vi "Adj Controls Pos.vi"(0 "Decoration Ref Array":refnum<vi>[](array[refnum]), 2 "Panel Bounds":T1, 5 "Add Display Ref (Bool)":refnum<vi>, 7 "Remove Display Ref (Bool)":refnum<vi>, 9 "Exit (Bool)":refnum<vi>, 11 "Message (String)":refnum<vi>, 12 "Max Left (Bool)":refnum<vi>, 13 "Max Right (Bool)":refnum<vi>) -> ()   [LabVIEW 2016]
uses:
  <vilib>/Utility/miscctls.llb/LVRectTypeDef.ctl
panel:
  in  "Add Display":bool
  in  "Remove Display":bool
  # "Copyright (C) 2020 Edward S Allgeyer\n\nRedistribution and use in source and binary forms, with or without\nmodification, are permitted provided that the following conditions\nare met:\n\n1. Redistributions of source code must retain the above copyright\n   notice, this list of conditions and the following disclaimer.\n\n2. Redistributions in binary form must reproduce the above copyright\n   notice, this list of conditions and the following disclaimer in\n   the documentation and/or other materials provided with the\n   distribution.\n\n3. Neither the name of the copyright holder nor the names of its\n   contributors may be used to endorse or promote products derived\n   from this software without specific prior written permission.\n\nTHIS SOFTWARE IS PROVIDED BY THE COPYRIGHT HOLDERS AND CONTRIBUTORS\n\"AS IS\" AND ANY EXPRESS OR IMPLIED WARRANTIES, INCLUDING, BUT NOT\nLIMITED TO, THE IMPLIED WARRANTIES OF MERCHANTABILITY AND FITNESS\nFOR A PARTICULAR PURPOSE ARE DISCLAIMED. IN NO EVENT SHALL THE\nCOPYRIGHT HOLDER OR CONTRIBUTORS BE LIABLE FOR ANY DIRECT, INDIRECT,\nINCIDENTAL, SPECIAL, EXEMPLARY, OR CONSEQUENTIAL DAMAGES (INCLUDING,\nBUT NOT LIMITED TO, PROCUREMENT OF SUBSTITUTE GOODS OR SERVICES;\nLOSS OF USE, DATA, OR PROFITS; OR BUSINESS INTERRUPTION) HOWEVER\nCAUSED AND ON ANY THEORY OF LIABILITY, WHETHER IN CONTRACT, STRICT\nLIABILITY, OR TORT (INCLUDING NEGLIGENCE OR OTHERWISE) ARISING IN\nANY WAY OUT OF THE USE OF THIS SOFTWARE, EVEN IF ADVISED OF THE\nPOSSIBILITY OF SUCH DAMAGE."
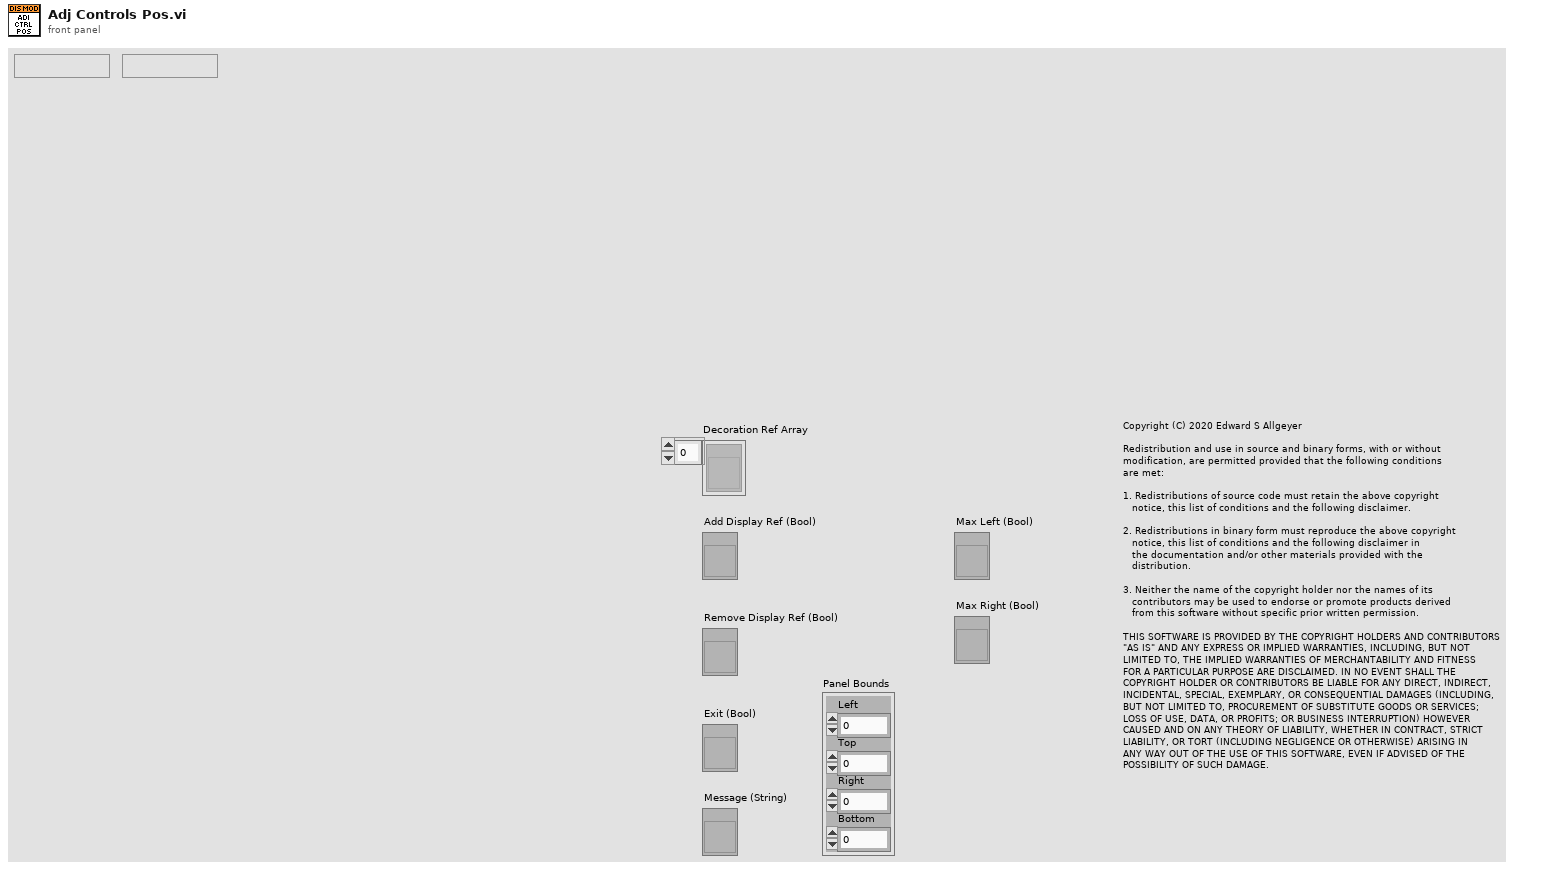
[diagram p1: front panel]
types:
  T1 = typedef "LVRectTypeDef.ctl" = cluster{"Left":i16, "Top":i16, "Right":i16, "Bottom":i16}
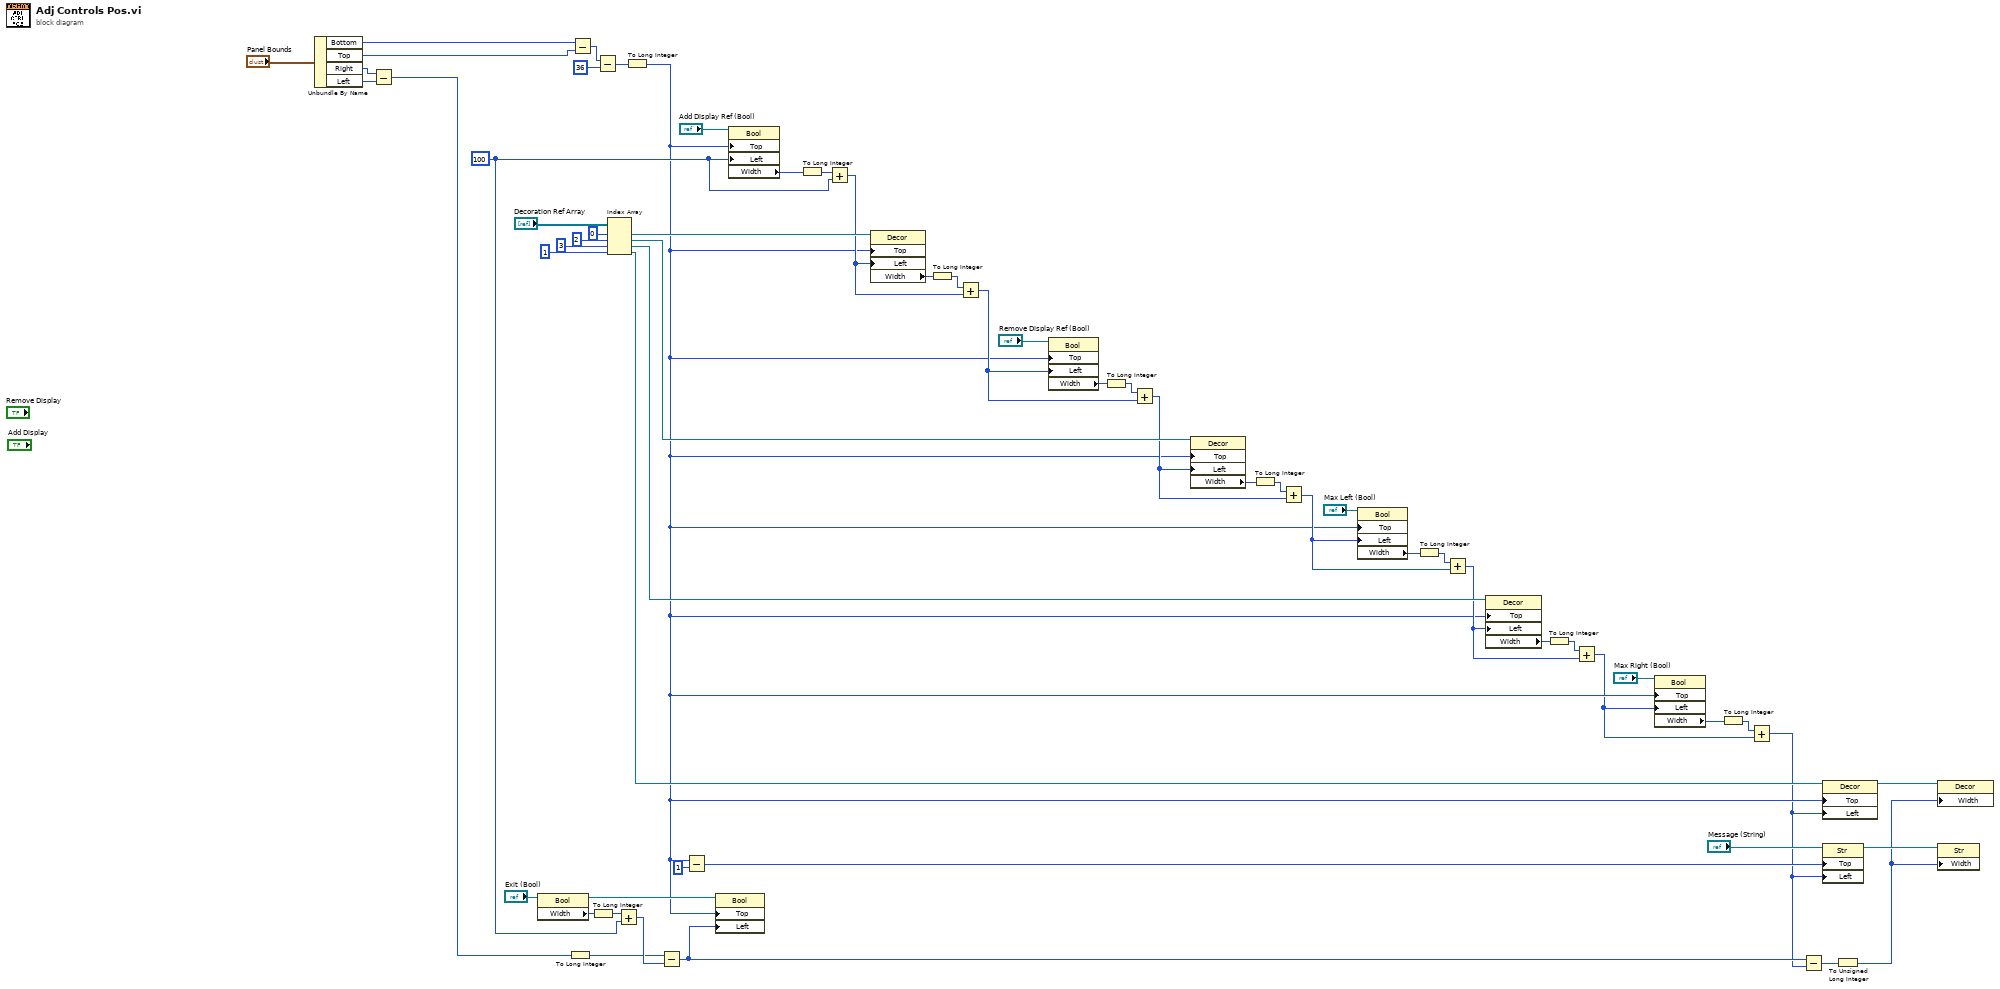
[diagram p0: block diagram]
diagram:
  w31 = 100 ("Position:Left")
  n1 = Unbundle By Name("Panel Bounds") -> ("Bottom"=w56:i16, "Top"=w55:i16, "Right"=w54:i16, "Left"=w53:i16)
  n2 = Subtract(x=w54, y=w53) -> (x-y=w29:i16)
  n3 = property class="Bool"(reference="Exit (Bool)") -> (reference out=w33:refnum<vi>, "Width"=w32:u32)  [unwired: 1 in, 1 out]
  n4 = To Long Integer(number=w29) -> (32bit integer=w27:i32)
  n5 = Subtract(x=w56, y=w55) -> (x-y=w59:i16)
  n6 = To Long Integer(number=w32) -> (32bit integer=w30:i32)
  n7 = Subtract(x=w59, y=i16 36) -> (x-y=w47:i16)
  n8 = Index Array(array="Decoration Ref Array", index #1=0 ("index"), index #2=2 ("index"), index #3=3 ("index"), index #4=1 ("index")) -> (element #1=w50:refnum<vi>, element #2=w17:refnum<vi>, element #3=w11:refnum<vi>, element #4=w19:refnum<vi>)
  n9 = Add(x=w30, y=w31) -> (x+y=w28:i32)
  n10 = To Long Integer(number=w47) -> (32bit integer=w5:i32)
  n11 = Subtract(x=w27, y=w28) -> (x-y=w24:i32)
  n12 = Subtract(x=w5, y=1) -> (x-y=w44:i32)
  n13 = property class="Bool"(reference=w33, "Top"=w5, "Left"=w24) -> ()  [unwired: 1 in, 2 out]
  n14 = property class="Bool"(reference="Add Display Ref (Bool)", "Top"=w5, "Left"=w31) -> ("Width"=w42:u32)  [unwired: 1 in, 2 out]
  n15 = To Long Integer(number=w42) -> (32bit integer=w41:i32)
  n16 = Add(x=w41, y=w31) -> (x+y=w36:i32)
  n17 = property class="Decor"(reference=w50, "Top"=w5, "Left"=w36) -> ("Width"=w40:u32)  [unwired: 1 in, 2 out]
  n18 = To Long Integer(number=w40) -> (32bit integer=w39:i32)
  n19 = Add(x=w39, y=w36) -> (x+y=w35:i32)
  n20 = property class="Bool"(reference="Remove Display Ref (Bool)", "Top"=w5, "Left"=w35) -> ("Width"=w37:u32)  [unwired: 1 in, 2 out]
  n21 = To Long Integer(number=w37) -> (32bit integer=w38:i32)
  n22 = Add(x=w38, y=w35) -> (x+y=w14:i32)
  n23 = property class="Decor"(reference=w17, "Top"=w5, "Left"=w14) -> ("Width"=w15:u32)  [unwired: 1 in, 2 out]
  n24 = To Long Integer(number=w15) -> (32bit integer=w16:i32)
  n25 = Add(x=w16, y=w14) -> (x+y=w10:i32)
  n26 = property class="Bool"(reference="Max Left (Bool)", "Top"=w5, "Left"=w10) -> ("Width"=w12:u32)  [unwired: 1 in, 2 out]
  n27 = To Long Integer(number=w12) -> (32bit integer=w13:i32)
  n28 = Add(x=w13, y=w10) -> (x+y=w7:i32)
  n29 = property class="Decor"(reference=w11, "Top"=w5, "Left"=w7) -> ("Width"=w8:u32)  [unwired: 1 in, 2 out]
  n30 = To Long Integer(number=w8) -> (32bit integer=w9:i32)
  n31 = Add(x=w9, y=w7) -> (x+y=w2:i32)
  n32 = property class="Bool"(reference="Max Right (Bool)", "Top"=w5, "Left"=w2) -> ("Width"=w3:u32)  [unwired: 1 in, 2 out]
  n33 = To Long Integer(number=w3) -> (32bit integer=w4:i32)
  n34 = Add(x=w4, y=w2) -> (x+y=w1:i32)
  n35 = Subtract(x=w24, y=w1) -> (x-y=w23:i32)
  n36 = property class="Decor"(reference=w19, "Top"=w5, "Left"=w1) -> (reference out=w26:refnum<vi>)  [unwired: 1 in, 1 out]
  n37 = property class="Str"(reference="Message (String)", "Top"=w44, "Left"=w1) -> (reference out=w25:refnum<vi>)  [unwired: 1 in, 1 out]
  n38 = To Unsigned Long Integer(number=w23) -> (unsigned 32bit integer=w22:u32)
  n39 = property class="Decor"(reference=w26, "Width"=w22) -> ()  [unwired: 1 in, 2 out]
  n40 = property class="Str"(reference=w25, "Width"=w22) -> ()  [unwired: 1 in, 2 out]
